vi "WPI_CANJaguar_UpdateSyncGroup.vi"(8 "error in (no error)":errorcluster, 9 "Sync Group":u8) -> (0 "error out":errorcluster)   [LabVIEW 2016]
doc: "When using CAN, this allows you to simultaneously update a group of motor controllers that were specified in the <B>WPI_MotorControlSetOutput</B> VI. This is a bitmask. When a value of 0 is used, this has no effect."
uses:
  <vilib>/Rock Robotics/WPI/CAN/Jaguar/SubVIs/WPI_CAN_SystemMessageIDs.ctl
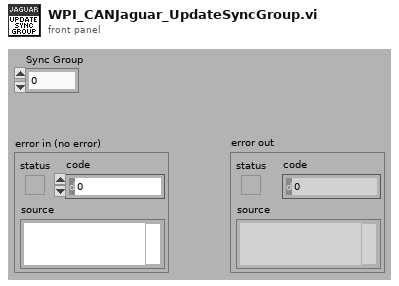
[diagram p1: front panel]
types:
  T1 = typedef "WPI_CAN_SystemMessageIDs.ctl" = u32
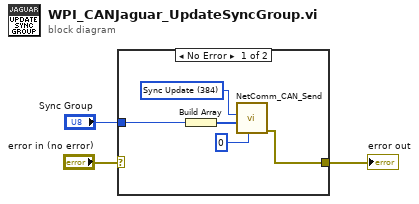
[diagram p0: block diagram]
diagram:
  n1 = case shown="No Error" "error in (no error)" {
    selector: "error in (no error)" -> [_ w9]
    tunnel: [w6 w9] -> w3
    tunnel: "Sync Group" -> [w8 _]
    frame No Error {
      w5 = T1 384 items=["Device Assignment"=128, "Device Query"=2147483840, "Sync Update"=384, "Firmware Update"=448, "Firmware Version"=2147484160, "Enumerate"=576] ("CAN System Message IDs")
      n2 = Build Array(w8) -> (w7:u8[])
      n3 = call <vilib>:"NetComm_CAN_Send.vi"("Period (ms)"=0, "Data"=w7, "Message ID"=w5) -> ("error out"=w6:errorcluster)  [unwired: 1 in, 7 out]
    }
    frame Error {
    }
  }
  "error out" <- w3
